vi "Import Serials Main.vi"() -> ()   [LabVIEW 2024]
uses:
  CTRLS/Open Batch Data.ctl
  <vilib>/Utility/miscctls.llb/LVPointTypeDef.ctl
  CTRLS/Serials DB Operations Enum.ctl
  CTRLS/GLB_VAR.vi
  <vilib>/Utility/file.llb/Read Delimited Spreadsheet (string).vi
panel:
  out "File Path":path
  in  "Batch Data":T1
  in  "Tab Control":enum32{"Page 1", "Page 2"}(tab)
  in  "Load CSV file":bool
  out "Title":string
  out "Import Result":string
  out "Batch File Found Message":string
  in  "Import Serials":bool
  out "Serials Found in File":dbl caption="Serial"
  in  "Close":bool
  in  "Directory path":path
  # "WO_Batch_GTIN_EXP_MFG"
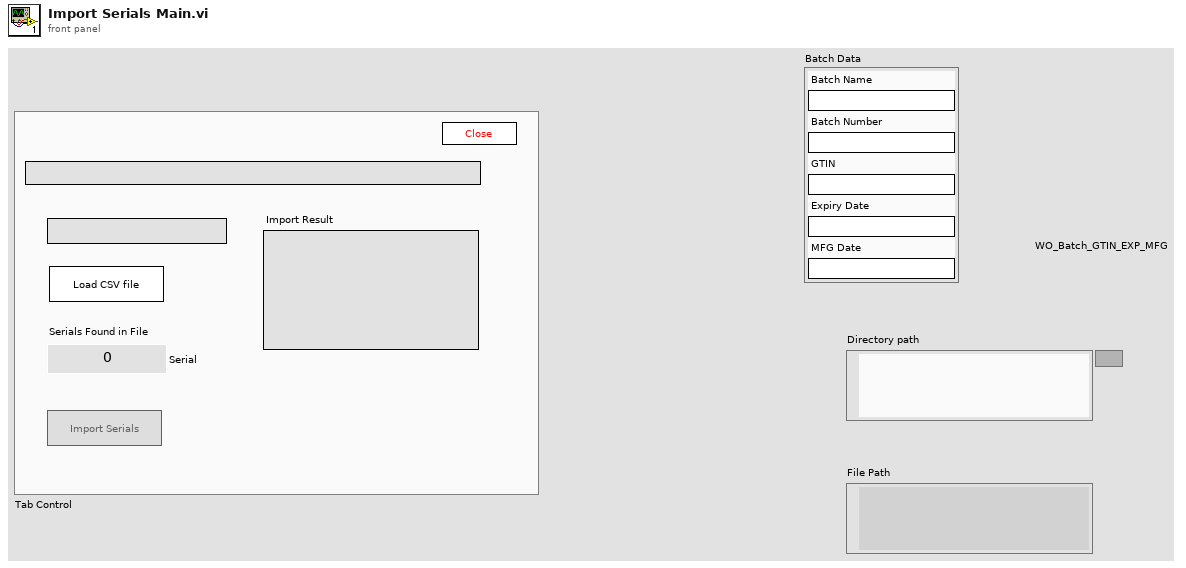
[diagram p1: front panel]
types:
  T1 = typedef "Open Batch Data.ctl" = cluster{"Batch Name":string, "Batch Number":string, "GTIN":string, "Expiry Date":string, "MFG Date":string}
  T2 = typedef "LVPointTypeDef.ctl" = cluster{"Horizontal":i16, "Vertical":i16}
  T3 = enum32{"Bad", "Idle", "Run top level", "Running"}
  T4 = typedef "REF.ctl" = cluster{"Save Settings":refnum<vi>, "Navigation":refnum<vi>, "Main Tab":refnum<vi>, "Password":refnum<vi>, "BatchData":refnum<vi>, "Serial Data":refnum<vi>, "Username":refnum<vi>, "Stop Printing":refnum<vi>, "Run statistics":refnum<vi>, "System settings":refnum<vi>, "Batch Managment contol":refnum<vi>, "Start Printing":refnum<vi>, "BatchData MNG":refnum<vi>, "MSG Cenetr":refnum<vi>, "Printer status":refnum<vi>, "Printer Message Config":refnum<vi>, "Ready and Paused Batches":refnum<vi>, "Camera Setup":refnum<vi>, "Batch statistics":refnum<vi>, "Logout":refnum<vi>}
  T5 = enum8{"Enabled", "Disabled", "Disabled and Grayed Out"}
  T6 = typedef "Serials DB Operations Enum.ctl" = enum16{"Update serial verify status", "Get serials Based on Status", "Insert serials", "Update serial print status", "Get all Batch Serials", "Get Serial Status"}
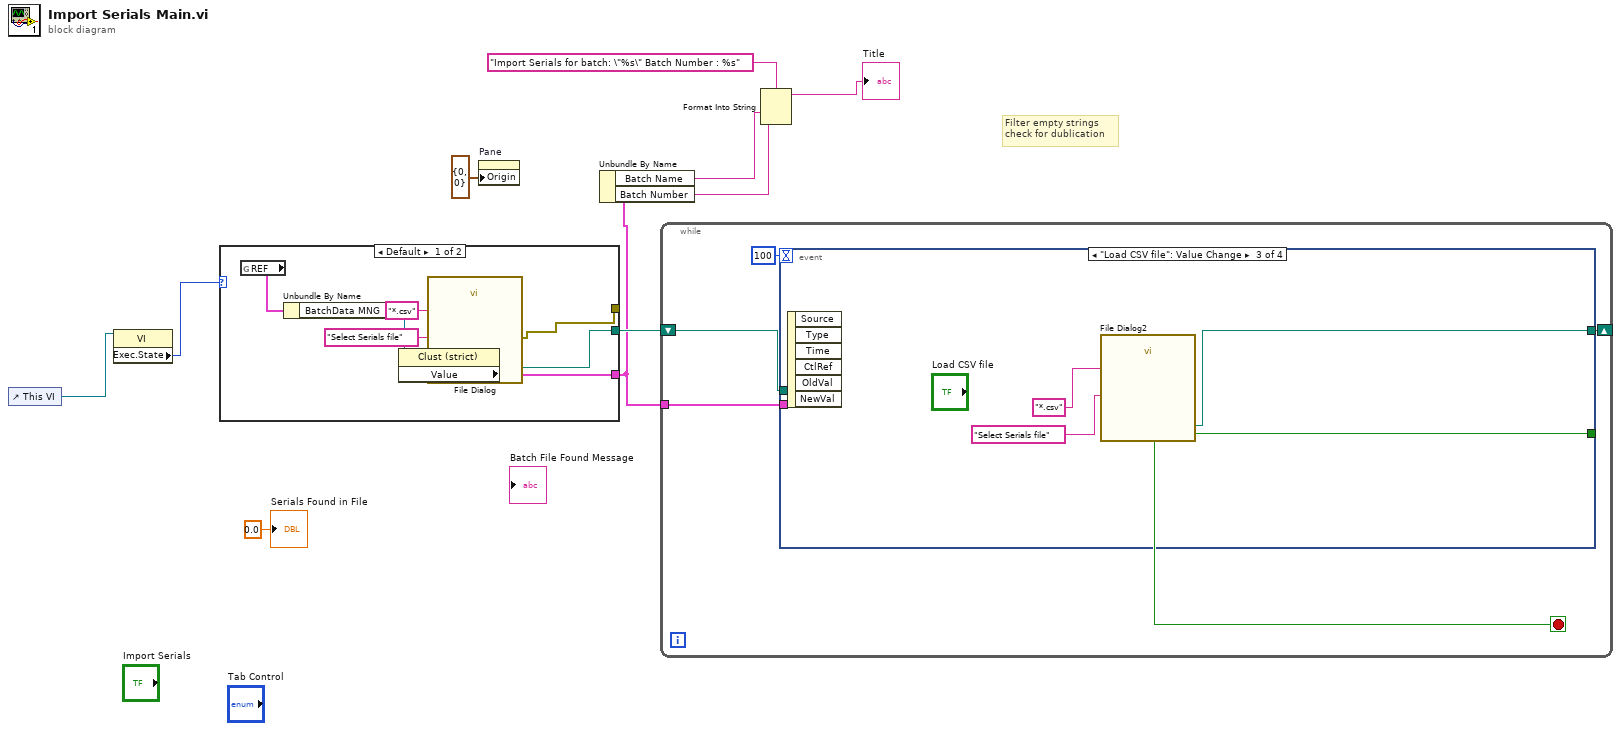
[diagram p0: block diagram]
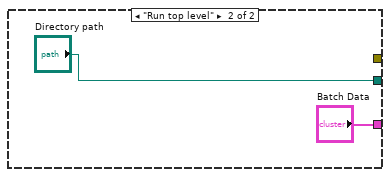
[diagram p2: hidden frame]
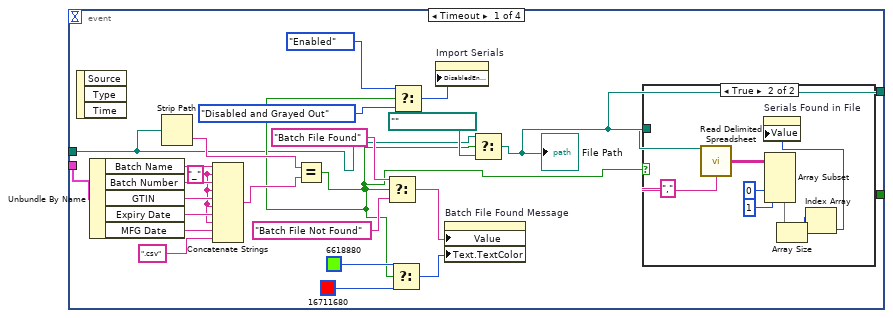
[diagram p3: hidden frame]
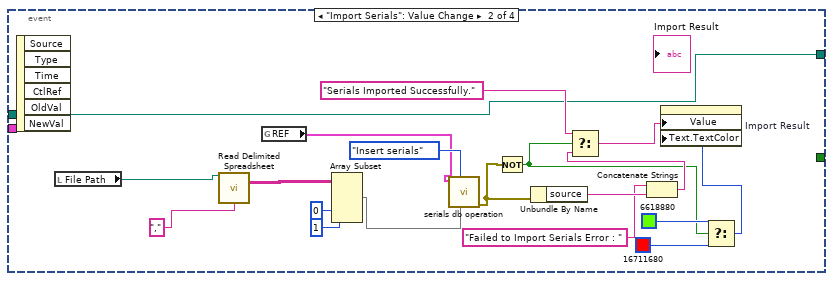
[diagram p5: hidden frame]
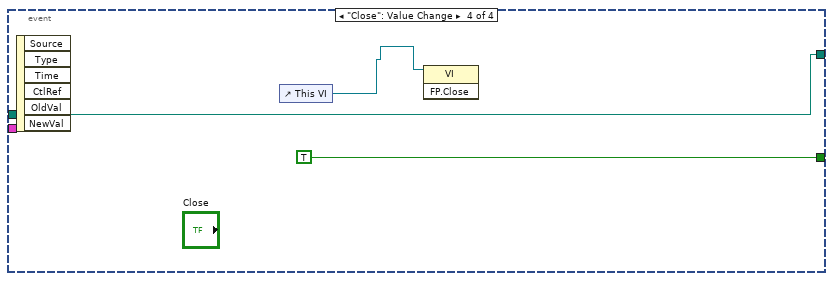
[diagram p6: hidden frame]
diagram:
  # "Filter empty strings\ncheck for dublication"
  n1 = control-ref of="This VI"() -> (w10:refnum<vi>)
  n2 = property class="VI"(reference=w10) -> ("Exec.State"=w9:T3)  [unwired: 1 in, 2 out]
  n3 = case shown="Default" w9 {
    tunnel: [w14 "Directory path"] -> w8
    tunnel: [w15 "Batch Data"] -> w6
    tunnel: [w11 _] -> _
    frame Default {
      n4 = global read "GLB_VAR.vi" "REF"() -> (w17:T4)
      n5 = Unbundle By Name(w17) -> ("BatchData MNG"=w16:refnum<vi>)
      n6 = property class="Clust (strict)"(reference=w16) -> ("Value"=w15:T1)  [unwired: 1 in, 2 out]
      n7 = call "File Dialog"("prompt"="Select Serials file", "pattern (all files)"="*.csv") -> ("selected path"=w14:path, "error out"=w11:errorcluster)  [unwired: 10 in, 2 out]
    }
    frame "Run top level" {
    }
  }
  n8 = property on="Pane" class="Pane"("Origin"=T2 {"Horizontal"=0, "Vertical"=0}) -> ()  [unwired: 2 in, 2 out]
  n9 = Unbundle By Name(w6) -> ("Batch Name"=w4:string, "Batch Number"=w3:string)
  n10 = while {
    tunnel: w6 -> [w21]
    shift-right: [w20] -> _
    shift-left: w8 -> [w22]
    stop <- w23 stop-if-true
    n11 = event shown="[2] \"Load CSV file\": Value Change" {
      selector: _ -> [_ _ _ _]
      dyn-events: _ -> [_ _ _ _]
      timeout: 100 -> [_ _ _ _]
      tunnel: [_ _ _ TRUE] -> w23
      tunnel: w22 -> [w26 w56 _ w78]
      tunnel: w21 -> [w47 _ _ _]
      tunnel: [w25 w56 w75 w78] -> w20
      event Timeout {
        w42 = "_" ("string")
        n12 = event-data() -> ()  [unwired: 1 in, 3 out]
        n13 = Unbundle By Name(w47) -> ("Batch Name"=w46:string, "Batch Number"=w45:string, "GTIN"=w44:string, "Expiry Date"=w43:string, "MFG Date"=w41:string)
        n14 = Strip Path(path=w26) -> (name=w29:string)  [unwired: 1 out]
        n15 = Concatenate Strings(w46, w42, w45, w42, w44, w42, w43, w42, w41, ".csv" ("string")) -> (w28:string)
        n16 = Equal?(x=w29, y=w28) -> (x = y?=w27:bool)
        n17 = Select(t="Batch File Found" ("string"), s=w27, f="Batch File Not Found" ("string")) -> (s? t:f=w34:string)
        n18 = Select(t=u32 6618880, s=w27, f=u32 16711680) -> (s? t:f=w35:u32)
        n19 = Select(t=T5."Enabled" ("Disabled"), s=w27, f=T5."Disabled and Grayed Out" ("Disabled")) -> (s? t:f=w31:T5)
        n20 = property on="Import Serials" class="Bool"("DisabledEnum"=w31) -> ()  [unwired: 2 in, 2 out]
        n21 = property on="Batch File Found Message" class="Str"("Value"=w34, "Text.TextColor"=w35) -> ()  [unwired: 2 in, 2 out]
        n22 = Select(t=w26, s=w27, f=path "" ("File Path")) -> (s? t:f=w25:path)
        "File Path" <- w25
        n23 = case shown="True" w27 {
          tunnel: w25 -> [_ w51]
          frame False {
          }
          frame True {
            n24 = call-poly <vilib>:"Read Delimited Spreadsheet.vi"("file path (dialog if empty)"=w51, "delimiter (\\t)"="," ("delimiter (\\t)")) -> ("all rows"=w53:string[][])  [unwired: 8 in, 5 out]
            n25 = Array Subset(array=w53, index (row)=1 ("index"), index (col)=0 ("index")) -> (w50:string[][])  [unwired: 2 in]
            n26 = Array Size(array=w50) -> (size(s)=w49:i32[])
            n27 = Index Array(array=w49) -> (element=w48:i32)  [unwired: 1 in]
            n28 = property on="Serials Found in File" class="DigNum (strict)"("Value"=w48) -> ()  [unwired: 2 in, 2 out]
          }
        }
      }
      event "Import Serials": Value Change {
        n29 = event-data() -> ()  [unwired: 1 in, 6 out]
        n30 = local read "File Path"() -> (w69:path)
        n31 = call-poly <vilib>:"Read Delimited Spreadsheet.vi"("file path (dialog if empty)"=w69, "delimiter (\\t)"="," ("delimiter (\\t)")) -> ("all rows"=w71:string[][])  [unwired: 8 in, 5 out]
        n32 = global read "GLB_VAR.vi" "REF"() -> (w67:T4)
        n33 = Array Subset(array=w71, index (row)=1 ("index"), index (col)=0 ("index")) -> (w74:string[][])  [unwired: 2 in]
        n34 = call "serials db operation.vi"("All serials Data"=w74, "SRL DB OP"=Serials_DB_Operations_Enum."Insert serials", "REF"=w67) -> ("error out"=w58:errorcluster)  [unwired: 5 in, 3 out]
        n35 = Not(x=w58) -> (.not. x?=w57:bool)
        n36 = Unbundle By Name(w58) -> ("source"=w65:string)
        n37 = Concatenate Strings("Failed to Import Serials Error : " ("delimiter (\\t)"), w65) -> (w63:string)
        n38 = Select(t="Serials Imported Successfully." ("delimiter (\\t)"), s=w57, f=w63) -> (s? t:f=w60:string)
        n39 = Select(t=u32 6618880, s=w57, f=u32 16711680) -> (s? t:f=w59:u32)
        n40 = property on="Import Result" class="Str"("Value"=w60, "Text.TextColor"=w59) -> ()  [unwired: 2 in, 2 out]
      }
      event "Load CSV file": Value Change {
        n41 = event-data() -> ()  [unwired: 1 in, 6 out]
        n42 = call "File Dialog2"("prompt"="Select Serials file", "pattern (all files)"="*.csv") -> ("selected path"=w75:path)  [unwired: 10 in, 3 out]
      }
      event "Close": Value Change {
        n43 = event-data() -> ()  [unwired: 1 in, 6 out]
        n44 = control-ref of="This VI"() -> (w79:refnum<vi>)
        n45 = invoke class="VI" method="FP.Close"(reference=w79) -> ()  [unwired: 2 in, 3 out]
      }
    }
  }
  n46 = Format Into String(format string="Import Serials for batch: \"%s\" Batch Number : %s", w4, w3) -> (resulting string=→"Title":string)  [unwired: 2 in, 1 out]
  "Serials Found in File" <- 0.0 ("Serials Found in File")
